vi "AVPP-constructor.vi"(8 "error in (no error)":errorcluster, 9 "FAMM.lvclass":refnum<class "FAMM.lvclass">, 10 "FAMM-Queue":refnum<queue>, 11 "AVPP in":refnum<class "AVPP.lvclass">) -> (0 "error out":errorcluster, 3 "AVPP out":refnum<class "AVPP.lvclass">)   [LabVIEW 2020, in "Sgraph_lib_V1.lvlib" / "AVPP.lvclass"]
doc: "Create AVPP object"
uses:
  AVPP.lvclass
  FAMM/controls/typedef_FAMM_Query.ctl
  FAMM/controls/typedef-functions.ctl
  FAMM/FAMM.lvclass
  AVPP.lvclass/AVPP.ctl
  Builds/Sgraph_lib_V1.lvlib
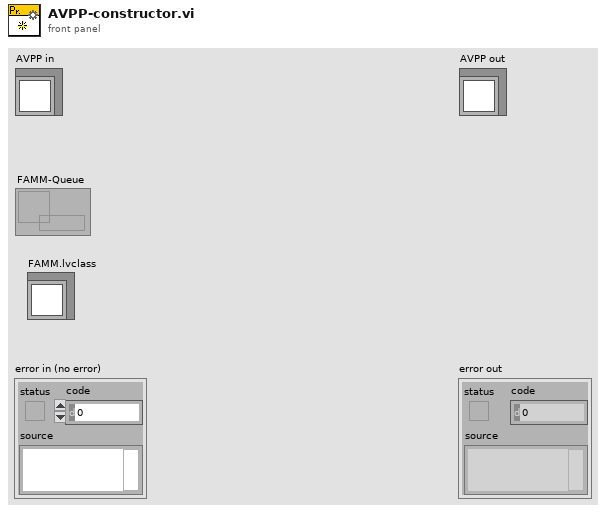
[diagram p1: front panel]
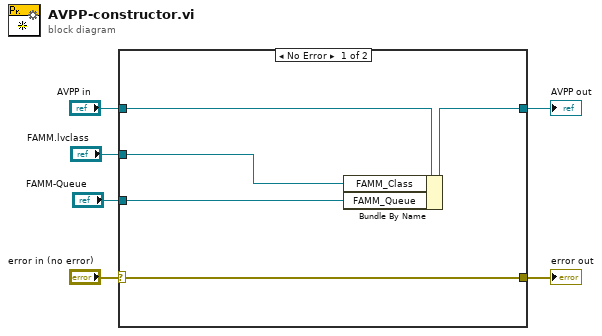
[diagram p0: block diagram]
diagram:
  n1 = case shown="No Error" "error in (no error)" {
    selector: "error in (no error)" -> [w9 w13]
    tunnel: [w9 w13] -> w5
    tunnel: [w10 w12] -> w3
    tunnel: "AVPP in" -> [w11 w12]
    tunnel: "FAMM-Queue" -> [w8 _]
    tunnel: "FAMM.lvclass" -> [w7 _]
    frame No Error {
      n2 = Bundle By Name(cluster=w11, "FAMM_Class"=w7, "FAMM_Queue"=w8) -> (w10:refnum<class "AVPP.lvclass">)
    }
    frame Error {
    }
  }
  "error out" <- w5
  "AVPP out" <- w3
